vi "Get Active Row.vi"(8 "error in (no error)":errorcluster caption="错误输入（无错误）", 9 "Vertical Position":i32 caption="垂直位置", 11 "Include Paths Ref":refnum<vi> caption="包括路径引用") -> (0 "error out":errorcluster caption="错误输出", 1 "Row Number":i32 caption="行数", 3 "Dup Include Paths Ref":refnum<vi> caption="包括路径引用副本")   [LabVIEW 2011, in "NISAST Include Paths.xctl"]
uses:
  NISAST Include Paths.xctl
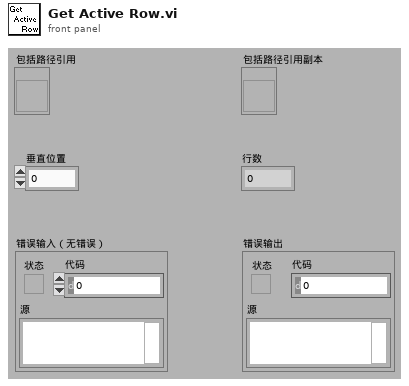
[diagram p1: front panel]
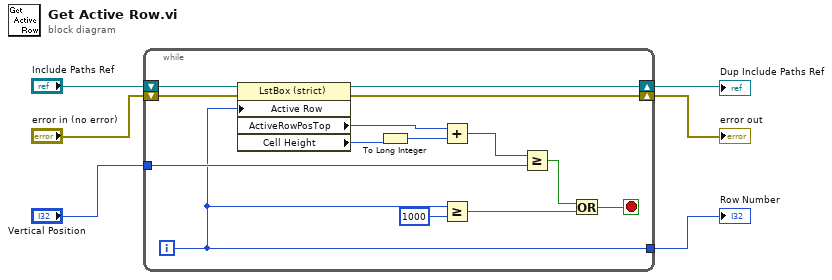
[diagram p0: block diagram]
diagram:
  n1 = while {
    tunnel: "Vertical Position" -> [w20]
    tunnel: [w7] -> w3
    shift-right: [w19] -> w2
    shift-left: "error in (no error)" -> [w8]
    shift-right: [w17] -> w1
    shift-left: "Include Paths Ref" -> [w9]
    i -> [w7]
    stop <- w10 stop-if-true
    n2 = property on="Property Node" class="LstBox (strict)"(reference=w9, error in=w8, "Active Row"=w7) -> (reference out=w17:refnum<vi>, error out=w19:errorcluster, "ActiveRowPosTop"=w18:i32, "Cell Height"=w16:i32)
    n3 = To Long Integer(number=w16) -> (32bit integer=w15:i32)
    n4 = Add(x=w18, y=w15) -> (x+y=w12:i32)
    n5 = Greater Or Equal?(x=w7, y=1000) -> (x >= y?=w14:bool)
    n6 = Greater Or Equal?(x=w12, y=w20) -> (x >= y?=w11:bool)
    n7 = Or(x=w11, y=w14) -> (x .or. y?=w10:bool)
  }
  "Row Number" <- w3
  "error out" <- w2
  "Dup Include Paths Ref" <- w1
